vi "API handler.vi"(8 "error in (no error)":errorcluster, 10 "user events":T1, 11 "Port (5555)":i32=5555) -> (0 "error out":errorcluster)   [LabVIEW 2020]
uses:
  user events.ctl
  api message.ctl
  api states.ctl
  <vilib>/addons/zeromq/socket_type.ctl
  global API.vi
  <vilib>/addons/zeromq/zeromq.lvlib
  <vilib>/addons/zeromq/zmq_context.lvclass
  <vilib>/addons/zeromq/zmq_socket.lvclass
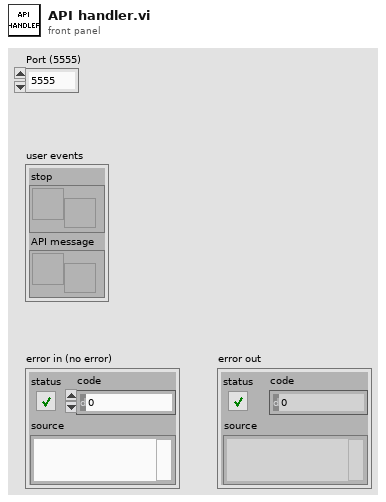
[diagram p1: front panel]
types:
  T1 = typedef "user events.ctl" = cluster{"stop":refnum<user-event>, "API message":refnum<user-event>}
  T2 = typedef "zeromq.lvlib/socket_type.ctl" = enum8{"ZMQ_PAIR", "ZMQ_PUB", "ZMQ_SUB", "ZMQ_REQ", "ZMQ_REP", "ZMQ_DEALER", "ZMQ_ROUTER", "ZMQ_PULL", "ZMQ_PUSH", "ZMQ_XPUB", "ZMQ_XSUB", "ZMQ_STREAM", "ZMQ_SERVER", "ZMQ_CLIENT", "ZMQ_RADIO", "ZMQ_DISH", "ZMQ_GATHER", "ZMQ_SCATTER", "ZMQ_DGRAM"}
  T3 = typedef "api message.ctl" = cluster{"API States":T4, "payload":variant}
  T4 = typedef "api states.ctl" = enum16{"stop", "say"}
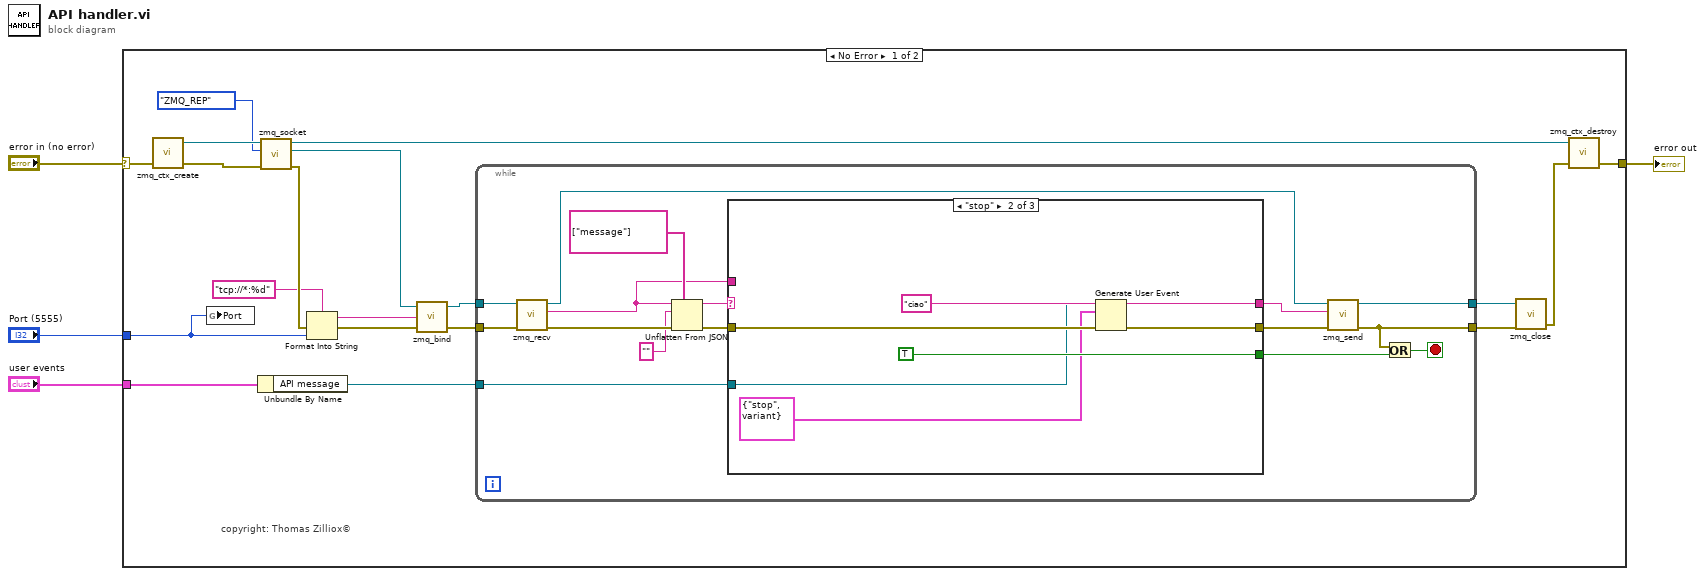
[diagram p0: block diagram]
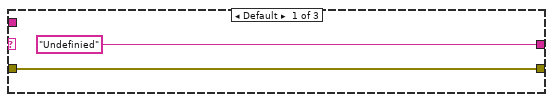
[diagram p2: hidden frame]
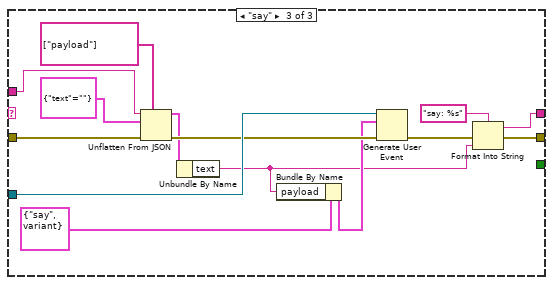
[diagram p3: hidden frame]
diagram:
  n1 = case shown="No Error" "error in (no error)" {
    selector: "error in (no error)" -> [w12 w62]
    tunnel: [w11 w62] -> w3
    tunnel: "Port (5555)" -> [w7 _]
    tunnel: "user events" -> [w6 _]
    frame No Error {
      # "copyright: Thomas Zilliox©"
      n2 = call <vilib>:"zmq_ctx_create.vi"("error in"=w12) -> ("error out"=w22:errorcluster, "context out"=w23:refnum<class "zmq_context.lvclass">)  [unwired: 3 in]
      n3 = global write "global API.vi" "Port"(w7) -> ()
      n4 = Unbundle By Name(w6) -> ("API message"=w5:refnum<user-event>)
      n5 = call <vilib>:"zmq_socket.vi"("error in"=w22, "socket type"=socket_type."ZMQ_REP", "context in"=w23) -> ("error out"=w18:errorcluster, "socket out"=w19:refnum<class "zmq_socket.lvclass">, "context out"=w20:refnum<class "zmq_context.lvclass">)  [unwired: 2 in]
      n6 = Format Into String(format string="tcp://*:%d" ("endpoint"), error in=w18, w7) -> (resulting string=w9:string, error out=w10:errorcluster)  [unwired: 1 in]
      n7 = call <vilib>:"zmq_bind.vi"("error in"=w10, "endpoint"=w9, "socket in"=w19) -> ("error out"=w16:errorcluster, "socket out"=w17:refnum<class "zmq_socket.lvclass">)  [unwired: 1 in]
      n8 = while {
        tunnel: w17 -> [w39]
        tunnel: w16 -> [w38]
        tunnel: [w36] -> w15
        tunnel: [w35] -> w14
        tunnel: w5 -> [w24]
        stop <- w34 stop-if-true
        n9 = call <vilib>:"zmq_recv.vi"("error in"=w38, "socket in"=w39) -> ("error out"=w31:errorcluster, "data"=w26:string, "socket out"=w37:refnum<class "zmq_socket.lvclass">)  [unwired: 3 in, 2 out]
        n10 = Unflatten From JSON(path=string[] ["message"], JSON string=w26, type and defaults="", error in (no error)=w31) -> (value=w28:string, error out=w30:errorcluster)  [unwired: 3 in]
        n11 = case shown="\"stop\"" w28 {
          tunnel: [w41 w44 w58] -> w33
          tunnel: w30 -> [w41 w47 w53]
          tunnel: [_ TRUE _] -> w32
          tunnel: ["Undefinied" ("data") "ciao" ("data") w56] -> w25
          tunnel: w26 -> [_ _ w48]
          tunnel: w24 -> [_ w43 w60]
          frame Default {
          }
          frame "stop" {
            n12 = Generate User Event(user event=w43, event data cluster=T3 {"API States"=enum."stop", "payload"=variant} ("event data"), error in=w47) -> (error out=w44:errorcluster)  [unwired: 1 in, 1 out]
          }
          frame "say" {
            n13 = Unflatten From JSON(path=string[] ["payload"], JSON string=w48, type and defaults=cluster{"text":string} {"text"=""}, error in (no error)=w53) -> (value=w51:cluster{"text":string}, error out=w52:errorcluster)  [unwired: 3 in]
            n14 = Unbundle By Name(w51) -> ("text"=w49:string)
            n15 = Bundle By Name(cluster=T3 {"API States"=enum."say", "payload"=variant} ("event data"), "payload"=w49) -> (w50:T3)
            n16 = Generate User Event(user event=w60, event data cluster=w50, error in=w52) -> (error out=w61:errorcluster)  [unwired: 1 in, 1 out]
            n17 = Format Into String(format string="say: %s" ("data"), error in=w61, w49) -> (resulting string=w56:string, error out=w58:errorcluster)  [unwired: 1 in]
          }
        }
        n18 = call <vilib>:"zmq_send.vi"("error in"=w33, "data"=w25, "socket in"=w37) -> ("error out"=w35:errorcluster, "socket out"=w36:refnum<class "zmq_socket.lvclass">)  [unwired: 4 in]
        n19 = Or(x=w35, y=w32) -> (x .or. y?=w34:bool)
      }
      n20 = call <vilib>:"zmq_close.vi"("error in"=w14, "socket"=w15) -> ("error out"=w13:errorcluster)  [unwired: 3 in]
      n21 = call <vilib>:"zmq_ctx_destroy.vi"("error in"=w13, "context in"=w20) -> ("error out"=w11:errorcluster)  [unwired: 3 in]
    }
    frame Error {
      # "copyright: Thomas Zilliox©"
    }
  }
  "error out" <- w3
